vi "Trim Whitespace__ogtk.vi"   [LabVIEW 2017]
doc: "Removes leading and/or trailing whitespace from a string.\nWhitespace is defined as any of the following characters (where values are in the format: dec, hex, string):\n <b>tab</b> = 9, 0x09, \\t\n <b>newline</b> = 10, 0x0A, \\n\n <b>vertical tab</b> = 11, 0x0B, \\0B\n <b>form feed</b> = 12, 0x0C, \\f\n <b>carriage return</b> = 13, 0x0D, \\r \n <b>space</b> = 32, 0x20, \\s"
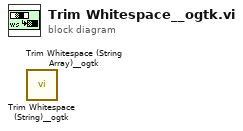
[diagram p0: block diagram]
diagram:
  n1 = call <userlib>:"Trim Whitespace (String)__ogtk.vi"() -> ()  [unwired: 7 in, 1 out]
  n2 = call <userlib>:"Trim Whitespace (String Array)__ogtk.vi"() -> ()  [unwired: 7 in, 1 out]
